vi "Update Plugin to Abort Name.vi"(8 "error in (no error)":errorcluster, 11 "CIF_UI in":refnum<class "CIF_UI.lvclass">) -> (0 "error out":errorcluster, 3 "CIF_UI out":refnum<class "CIF_UI.lvclass">)   [LabVIEW 2021, in "CIF_UI.lvclass"]
uses:
  CIF_UI.lvclass
  CIF_UI.lvclass/CIF_UI.ctl
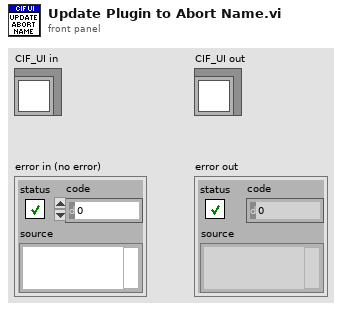
[diagram p1: front panel]
types:
  T1 = typedef "CIF_UI.lvclass/Plugin Connection Map.ctl" = map{string, T2}
  T2 = typedef "CIF_UI.lvclass/Plugin Connections.ctl" = cluster{"gRPC ID":T3, "Plugin info":T4}
  T3 = typedef "grpc-lvsupport-release.lvlib/grpcId.ctl" = u64
  T4 = typedef "CIF_Manager_client.lvlib/cif_manager_PluginInfo.ctl" = cluster{"plugin_name":string, "plugin_type":string, "grpc_port":i32, "plugin_version":T5, "status":T6}
  T5 = typedef "CIF_Manager_client.lvlib/cif_manager_PluginVersion.ctl" = cluster{"major_version":i32, "minor_version":i32, "fix_version":i32, "build_version":i32}
  T6 = typedef "CIF_Manager_client.lvlib/cif_plugincore_StatusData.ctl" = cluster{"state":T7, "timing_statistics":T8, "fifo_statistics":T10, "error":T11, "monitor_doubles":T12, "monitor_u64s":T13, "monitor_i64s":T14}
  T7 = typedef "CIF_Manager_client.lvlib/cif_plugincore_StatusData_State.ctl" = enum32{"NULL", "CREATING", "LISTENING", "RUNNING", "CLEANINGUP", "DESTROYING"}
  T8 = typedef "CIF_Manager_client.lvlib/cif_plugincore_TimingStatistics.ctl" = cluster{"period":T9, "wake_error":T9, "execute":T9, "housekeep":T9, "idle":T9}
  T9 = typedef "CIF_Manager_client.lvlib/cif_plugincore_TimingStatsBasic.ctl" = cluster{"max":i32, "min":i32}
  T10 = typedef "CIF_Manager_client.lvlib/cif_plugincore_FifoStatistics.ctl" = cluster{"from_t0":T9, "from_previous_plugin":T9, "output_error":T9}
  T11 = typedef "CIF_Manager_client.lvlib/cif_plugincore_Error.ctl" = cluster{"status":bool, "code":i32}
  T12 = typedef "CIF_Manager_client.lvlib/cif_plugincore_MonitorDoubles.ctl" = cluster{"double_1":dbl, "double_2":dbl, "double_3":dbl, "double_4":dbl}
  T13 = typedef "CIF_Manager_client.lvlib/cif_plugincore_MonitorU64.ctl" = cluster{"u64_1":u64, "u64_2":u64, "u64_3":u64, "u64_4":u64}
  T14 = typedef "CIF_Manager_client.lvlib/cif_plugincore_MonitorI64.ctl" = cluster{"i64_1":i64, "i64_2":i64, "i64_3":i64, "i64_4":i64}
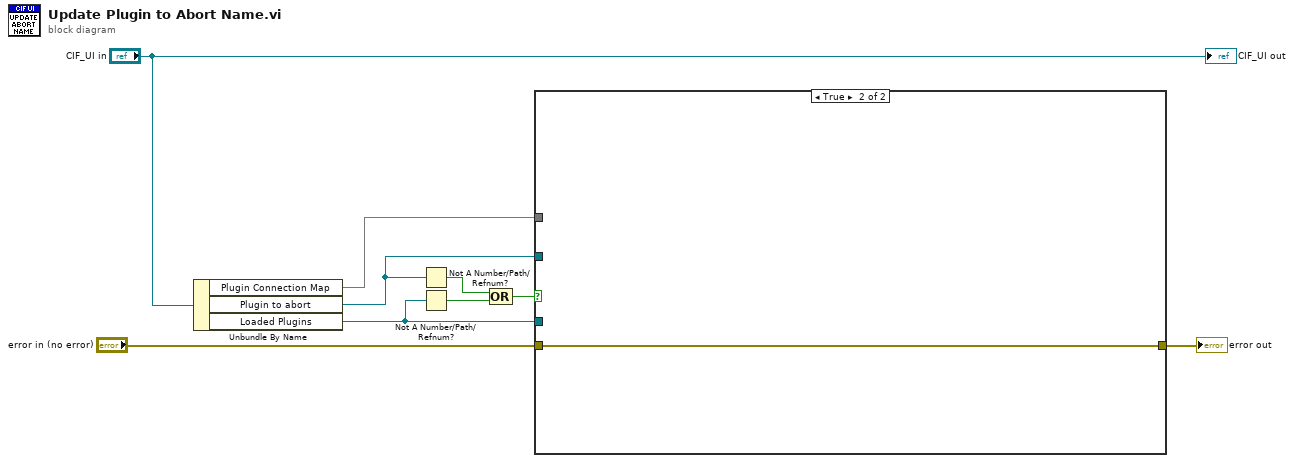
[diagram p0: block diagram]
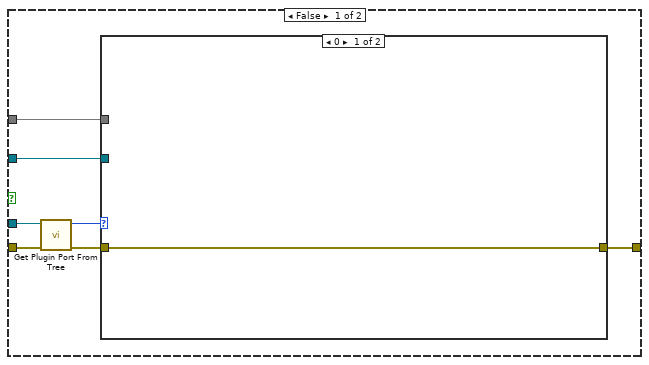
[diagram p2: hidden frame]
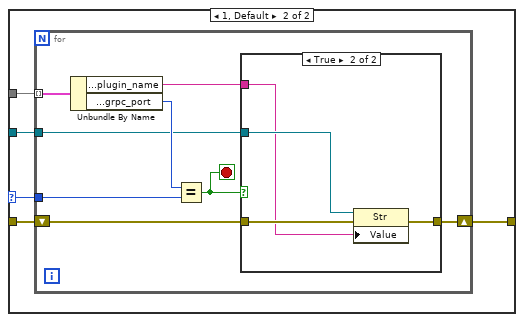
[diagram p3: hidden frame]
diagram:
  n1 = Unbundle By Name("CIF_UI in") -> ("Plugin Connection Map"=w9:T1, "Plugin to abort"=w7:refnum<vi>, "Loaded Plugins"=w6:refnum<vi>)
  n2 = Not A Number/Path/Refnum?(number/path/refnum=w7) -> (NaN/Path/Refnum?=w4:bool)
  n3 = Not A Number/Path/Refnum?(number/path/refnum=w6) -> (NaN/Path/Refnum?=w5:bool)
  n4 = Compound Arithmetic op=OR(w4, w5) -> (w3:bool)
  n5 = case shown="True" w3 {
    tunnel: w9 -> [w16 _]
    tunnel: "error in (no error)" -> [w15 w36]
    tunnel: w7 -> [w14 _]
    tunnel: w6 -> [w13 _]
    tunnel: [w10 w36] -> w2
    frame False {
      n6 = call "Get Plugin Port From Tree.vi"("error in (no error)"=w15, "Loaded Plugins"=w13) -> ("error out"=w12:errorcluster, "Plugin port"=w11:i32)  [unwired: 8 in]
      n7 = case shown="0" w11 {
        selector: w11 -> [_ w19]
        tunnel: w16 -> [_ w22]
        tunnel: w14 -> [_ w21]
        tunnel: w12 -> [w17 w20]
        tunnel: [w17 w18] -> w10
        frame 0 {
        }
        frame 1, Default {
          n8 = for {
            tunnel: w22 -> [w30] mode=indexing
            tunnel: w19 -> [w29]
            tunnel: w21 -> [w25]
            shift-right: [w23] -> w18
            shift-left: w20 -> [w24]
            stop <- w27 stop-if-true
            n9 = Unbundle By Name(w30) -> ("Plugin Connections.Plugin info.plugin_name"=w26:string, "Plugin Connections.Plugin info.grpc_port"=w28:i32)
            n10 = Equal?(x=w28, y=w29) -> (x = y?=w27:bool)
            n11 = case shown="True" w27 {
              tunnel: w26 -> [_ w33]
              tunnel: w25 -> [_ w34]
              tunnel: w24 -> [w31 w35]
              tunnel: [w31 w32] -> w23
              frame False {
              }
              frame True {
                n12 = property class="Str"(reference=w34, error in=w35, "Value"=w33) -> (error out=w32:errorcluster)  [unwired: 1 out]
              }
            }
          }
        }
      }
    }
    frame True {
    }
  }
  "error out" <- w2
  "CIF_UI out" <- "CIF_UI in"
